vi "TestInterface.vi"() -> ()   [LabVIEW 2017]
uses:
  <vilib>/Instr/_visa.llb/VISA Configure Serial Port (Instr).vi
panel:
  out "string":string
  in  "VISA resource name":refnum<visa-resource-name>="COM4"
  in  "Steering":u8(slide)=90 scale=0.0..120.0
  in  "Throttle":u8(slide)=90 scale=0.0..180.0
  in  "stop":bool
  in  "Numeric":u8
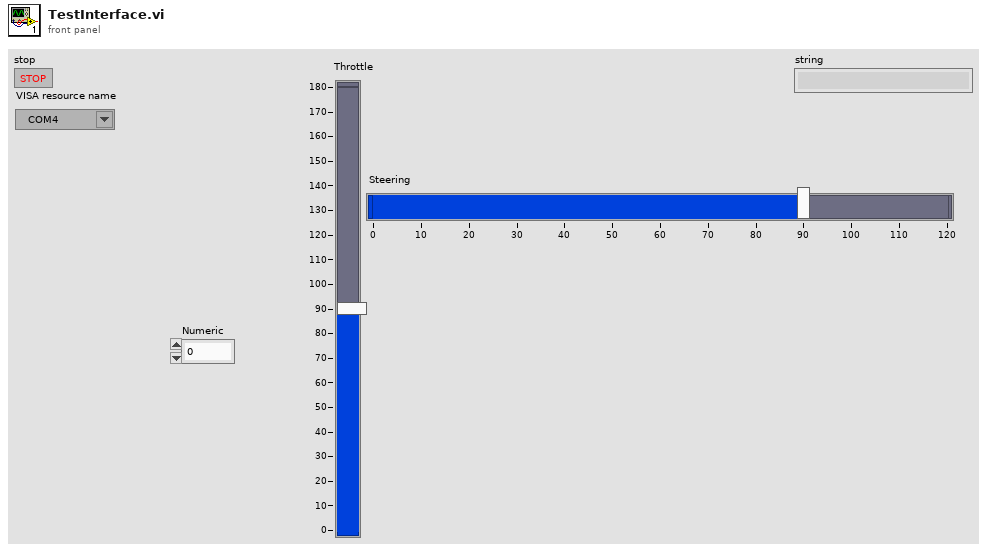
[diagram p1: front panel]
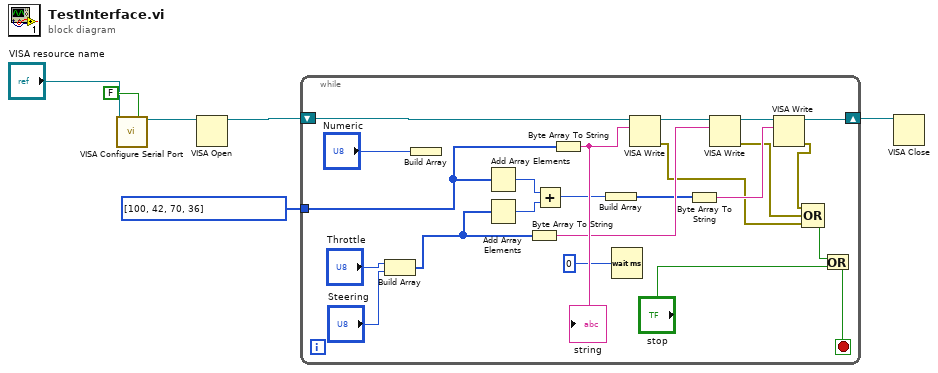
[diagram p0: block diagram]
diagram:
  n1 = call-poly "VISA Configure Serial Port"("VISA resource name"="VISA resource name", "Enable Termination\nChar (T)"=FALSE ("Enable Termination\nChar (T)")) -> ("VISA resource name out"=w2:refnum<visa-resource-name>)  [unwired: 12 in, 1 out]
  n2 = VISA Open(VISA resource name=w2) -> (VISA resource name=w5:refnum<visa-resource-name>)  [unwired: 4 in, 1 out]
  n3 = while {
    shift-right: [w14] -> w4
    shift-left: w5 -> [w29]
    tunnel: u8[] [100, 42, 70, 36] -> [w19]
    stop <- w25 stop-if-true
    n4 = Build Array("Throttle", "Steering") -> (w18:u8[])
    n5 = Build Array("Numeric") -> ()  [unwired: 1 out]
    n6 = Add Array Elements(numeric array=w19) -> (sum=w17:u8)
    n7 = Add Array Elements(numeric array=w18) -> (sum=w16:u8)
    n8 = Byte Array To String(unsigned byte array=w18) -> (string=w20:string)
    n9 = Add(x=w17, y=w16) -> (x+y=w13:u8)
    n10 = Byte Array To String(unsigned byte array=w19) -> (string=w27:string)
    "string" <- w27
    n11 = Build Array(w13) -> (w12:u8[])
    n12 = Wait (ms)(milliseconds to wait=u32 0) -> ()  [unwired: 1 out]
    n13 = VISA Write(VISA resource name=w29, write buffer=w27) -> (VISA resource name out=w21:refnum<visa-resource-name>, error out=w8:errorcluster)  [unwired: 1 in, 1 out]
    n14 = Byte Array To String(unsigned byte array=w12) -> (string=w11:string)
    n15 = VISA Write(VISA resource name=w21, write buffer=w20) -> (VISA resource name out=w15:refnum<visa-resource-name>, error out=w9:errorcluster)  [unwired: 1 in, 1 out]
    n16 = VISA Write(VISA resource name=w15, write buffer=w11) -> (VISA resource name out=w14:refnum<visa-resource-name>, error out=w10:errorcluster)  [unwired: 1 in, 1 out]
    n17 = Compound Arithmetic op=OR(w10, w9, w8) -> (w7:bool)
    n18 = Or(x=w7, y="stop") -> (x .or. y?=w25:bool)
  }
  n19 = VISA Close(VISA resource name=w4) -> ()  [unwired: 1 in, 1 out]
